vi "Actor Core.vi"(8 "error in":errorcluster caption="错误输入", 11 "服务器":refnum<class "服务器.lvclass"> caption="操作者输入") -> (0 "error out":errorcluster caption="错误输出", 3 "Actor out":refnum<class "Actor.lvclass"> caption="操作者输出")   [LabVIEW 2015, in "服务器.lvlib" / "服务器.lvclass"]
doc: "(<B>Filename</B>: Actor Framework.lvlib:Actor.lvclass:Actor Core.vi)\n\nReceives messages to the actor, reacts to them, and initiates any error handling that may shut the actor down.\n\nDescendant classes may override this VI to append parallel tasks for the actor to complete while it handles messages. Overrides use the Call Parent Method node."
uses:
  <vilib>/ActorFramework/Actor/Actor.lvclass
  <vilib>/ActorFramework/Stop Msg/Stop Msg.lvclass
  <vilib>/Instr/_visa.llb/VISA Configure Serial Port (Instr).vi
panel:
  in  "打开下位机":bool
  in  "控制中心":i32(listbox)
  in  "停止按钮":bool
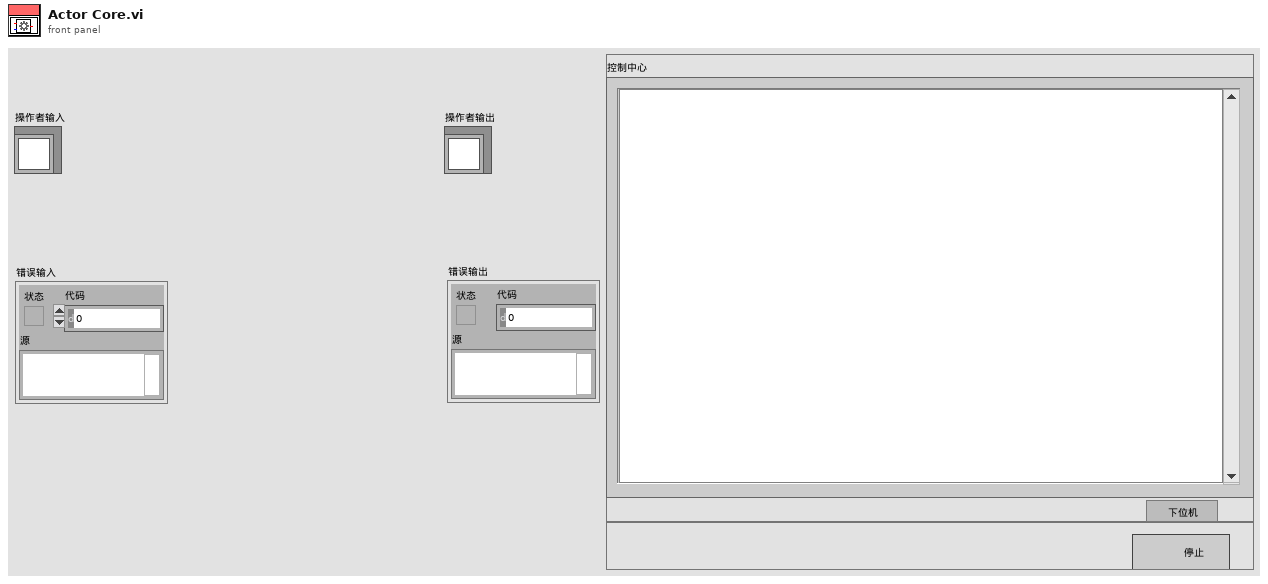
[diagram p1: front panel]
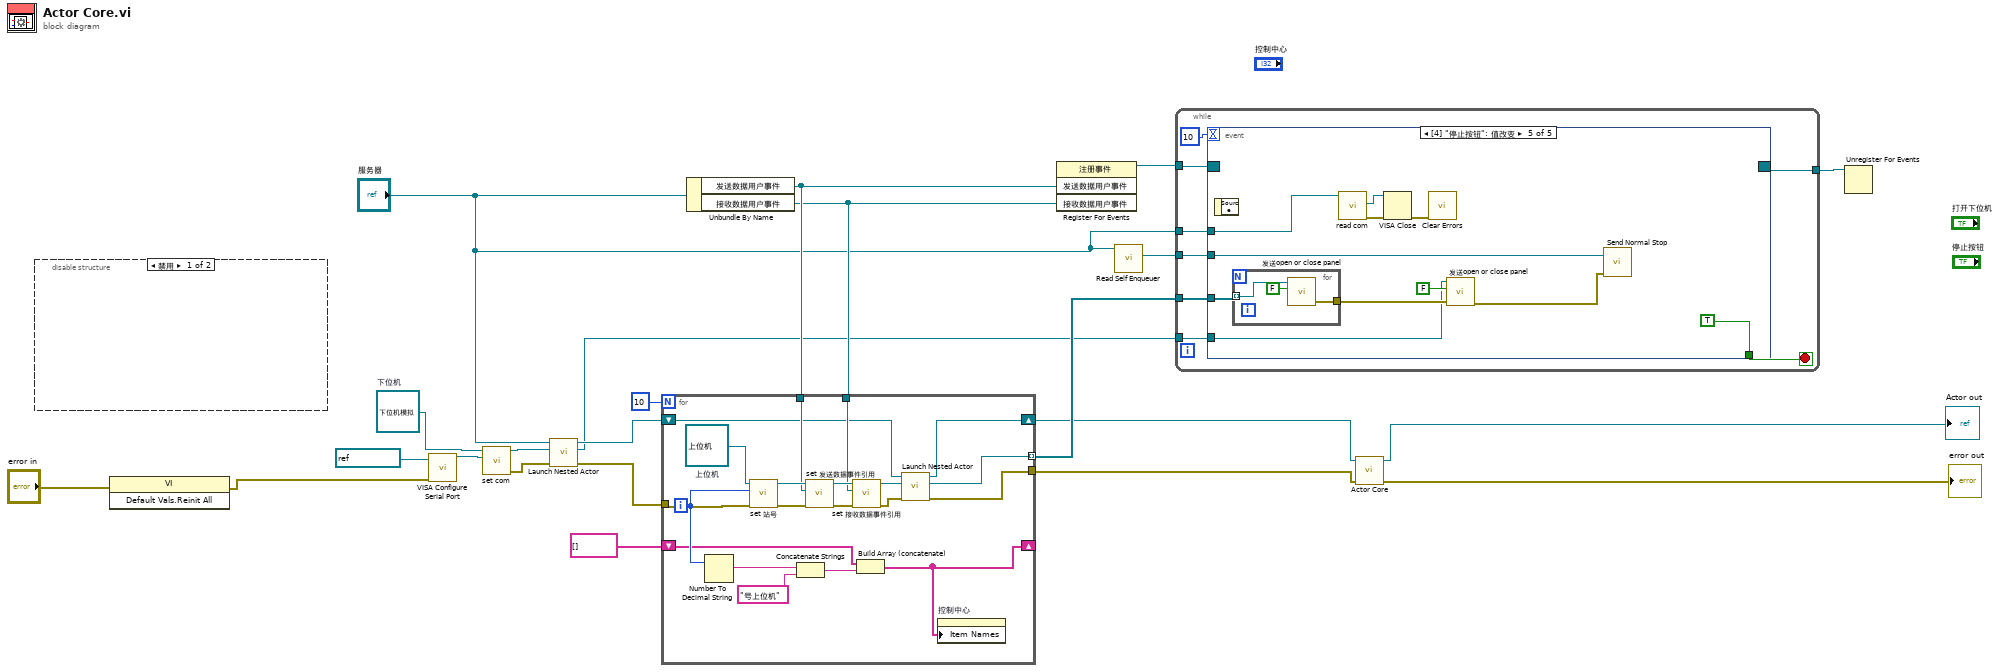
[diagram p0: block diagram]
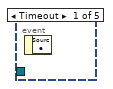
[diagram p3: hidden frame]
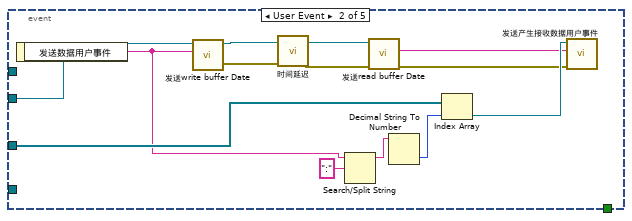
[diagram p4: hidden frame]
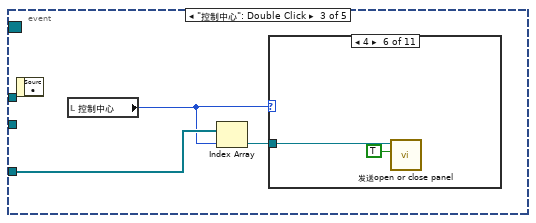
[diagram p5: hidden frame]
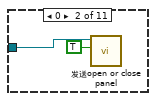
[diagram p7: hidden frame]
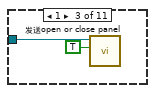
[diagram p8: hidden frame]
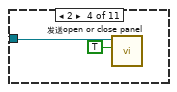
[diagram p9: hidden frame]
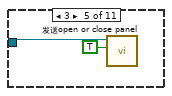
[diagram p10: hidden frame]
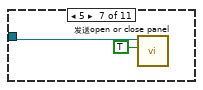
[diagram p11: hidden frame]
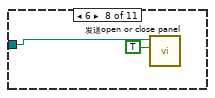
[diagram p12: hidden frame]
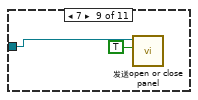
[diagram p13: hidden frame]
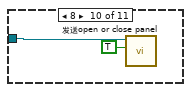
[diagram p14: hidden frame]
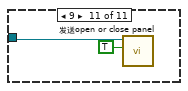
[diagram p15: hidden frame]
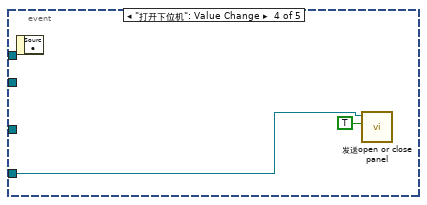
[diagram p16: hidden frame]
diagram:
  w10 = refnum<class "下位机模拟.lvclass"> refnum  # 下位机
  n1 = disable-structure shown="禁用" {
    frame Disabled {
    }
    frame Enabled {
    }
  }
  n2 = invoke class="VI" method="Default Vals.Reinit All"(error in="error in") -> (error out=w6:errorcluster)  [unwired: 2 in, 2 out]
  n3 = call-poly "VISA Configure Serial Port"("VISA resource name"=refnum<visa-resource-name> "COM29", "error in (no error)"=w6) -> ("VISA resource name out"=w7:refnum<visa-resource-name>)  [unwired: 12 in, 1 out]
  n4 = call "set com.vi"("COM"=w7, "串口参数管理 输入"=w10) -> ("error out"=w9:errorcluster, "串口参数管理 输出"=w11:refnum<class "下位机模拟.lvclass">)  [unwired: 8 in]
  n5 = call <vilib>:"Launch Nested Actor.vi"("error in (no error)"=w9, "Nested Actor"=w11, "Caller Actor in"="服务器") -> ("error out"=w4:errorcluster, "Nested Actor's Enqueuer"=w1:refnum<class "Message Enqueuer.lvclass">, "Caller Actor out"=w3:refnum<class "服务器.lvclass">)  [unwired: 6 in]
  n6 = Unbundle By Name("服务器") -> ("发送数据用户事件"=w18:refnum<user-event>, "接收数据用户事件"=w17:refnum<user-event>)
  n7 = for {
    N: 10 -> [_]
    tunnel: [w43] -> w22 mode=indexing
    tunnel: w18 -> [w36]
    tunnel: w17 -> [w35]
    tunnel: [w34] -> w13
    shift-right: [w28] -> _
    shift-left: string[] [] ("项名") -> [w27]
    tunnel: w4 -> [w26]
    shift-right: [w24] -> w2
    shift-left: w3 -> [w25]
    i -> [w30]
    w31 = refnum<class "上位机.lvclass"> refnum  # 上位机
    n8 = Number To Decimal String(number=w30) -> (decimal integer string=w29:string)  [unwired: 1 in]
    n9 = call "set 站号.vi"("error in (no error)"=w26, "站号"=w30, "上位机 输入"=w31) -> ("error out"=w39:errorcluster, "上位机 输出"=w42:refnum<class "上位机.lvclass">)  [unwired: 7 in]
    n10 = Concatenate Strings(w29, "号上位机" ("字符串")) -> (w32:string)
    n11 = call "set 发送数据事件引用.vi"("error in (no error)"=w39, "发送数据用户事件"=w36, "上位机 输入"=w42) -> ("error out"=w38:errorcluster, "上位机 输出"=w41:refnum<class "上位机.lvclass">)  [unwired: 7 in]
    n12 = call "set 接收数据事件引用.vi"("error in (no error)"=w38, "接收数据用户事件"=w35, "上位机 输入"=w41) -> ("error out"=w37:errorcluster, "上位机 输出"=w40:refnum<class "上位机.lvclass">)  [unwired: 7 in]
    n13 = Build Array (concatenate)(w27, w32) -> (w28:string[])
    n14 = call <vilib>:"Launch Nested Actor.vi"("error in (no error)"=w37, "Nested Actor"=w40, "Caller Actor in"=w25) -> ("error out"=w34:errorcluster, "Nested Actor's Enqueuer"=w43:refnum<class "Message Enqueuer.lvclass">, "Caller Actor out"=w24:refnum<class "服务器.lvclass">)  [unwired: 6 in]
    n15 = property on="控制中心" class="LstBox (严格)"("Item Names"=w28) -> ()  [unwired: 2 in, 2 out]
  }
  n16 = register-events(w18, w17) -> (reference out=w21:refnum<event-registration>)  [unwired: 2 in, 1 out]
  n17 = call <vilib>:"Read Self Enqueuer.vi"("Actor"="服务器") -> ("Self Enqueuer"=w15:refnum<class "Message Enqueuer.lvclass">)  [unwired: 10 in]
  n18 = while {
    tunnel: w22 -> [w49]
    tunnel: w21 -> [w51]
    tunnel: [w50] -> w20
    tunnel: w15 -> [w46]
    tunnel: "服务器" -> [w45]
    tunnel: w1 -> [w44]
    stop <- w48 stop-if-true
    n19 = event shown="[4] \"停止按钮\": 值改变" {
      selector: w51 -> [_ _ _ _ _]
      dyn-events: [_ _ _ _ _] -> w50
      timeout: 10 -> [_ _ _ _ _]
      tunnel: w49 -> [_ w60 w66 _ w93]
      tunnel: [_ _ _ _ TRUE] -> w48
      tunnel: w46 -> [_ w58 _ _ w95]
      tunnel: w45 -> [_ _ _ _ w94]
      tunnel: w44 -> [_ _ _ w87 w89]
      event Timeout {
        n20 = event-data() -> ()  [unwired: 1 in, 1 out]
      }
      event User Event {
        n21 = event-data() -> ("发送数据用户事件"=w57:string)  [unwired: 1 in]
        n22 = call "发送write buffer Date.vi"("写入缓冲区"=w57, "Message Enqueuer"=w58) -> ("error out"=w56:errorcluster, "Message Enqueuer out"=w55:refnum<class "Message Enqueuer.lvclass">)  [unwired: 8 in]
        n23 = call "时间延迟"("error in (no error)"=w56) -> ("error out"=w54:errorcluster)  [unwired: 10 in]
        n24 = Search/Split String(string=w57, search string/char (-)=":") -> (substring before match=w63:string)  [unwired: 1 in, 2 out]
        n25 = call "发送read buffer Date.vi"("error in (no error)"=w54, "Message Enqueuer"=w55) -> ("error out"=w53:errorcluster, "read buffer date"=w52:string)  [unwired: 7 in, 1 out]
        n26 = Decimal String To Number(string=w63) -> (number=w62:i32)  [unwired: 2 in, 1 out]
        n27 = Index Array(array=w60, index=w62) -> (element=w59:refnum<class "Message Enqueuer.lvclass">)
        n28 = call "发送产生接收数据用户事件.vi"("error in (no error)"=w53, "产生接收数据事件"=w52, "Message Enqueuer"=w59) -> ()  [unwired: 7 in, 2 out]
      }
      event "控制中心": Double Click {
        n29 = event-data() -> ()  [unwired: 1 in, 1 out]
        n30 = local read "控制中心"() -> (w65:i32)
        n31 = Index Array(array=w66, index=w65) -> (element=w64:refnum<class "Message Enqueuer.lvclass">)
        n32 = case shown="4" w65 {
          tunnel: w64 -> [_ w68 w70 w72 w73 w75 w77 w79 w81 w83 w85]
          frame Default {
          }
          frame 0 {
            n33 = call "发送open or close panel.vi"("布尔"=TRUE, "Message Enqueuer"=w68) -> ()  [unwired: 8 in, 2 out]
          }
          frame 1 {
            n34 = call "发送open or close panel.vi"("布尔"=TRUE, "Message Enqueuer"=w70) -> ()  [unwired: 8 in, 2 out]
          }
          frame 2 {
            n35 = call "发送open or close panel.vi"("布尔"=TRUE, "Message Enqueuer"=w72) -> ()  [unwired: 8 in, 2 out]
          }
          frame 3 {
            n36 = call "发送open or close panel.vi"("布尔"=TRUE, "Message Enqueuer"=w73) -> ()  [unwired: 8 in, 2 out]
          }
          frame 4 {
            n37 = call "发送open or close panel.vi"("布尔"=TRUE, "Message Enqueuer"=w75) -> ()  [unwired: 8 in, 2 out]
          }
          frame 5 {
            n38 = call "发送open or close panel.vi"("布尔"=TRUE, "Message Enqueuer"=w77) -> ()  [unwired: 8 in, 2 out]
          }
          frame 6 {
            n39 = call "发送open or close panel.vi"("布尔"=TRUE, "Message Enqueuer"=w79) -> ()  [unwired: 8 in, 2 out]
          }
          frame 7 {
            n40 = call "发送open or close panel.vi"("布尔"=TRUE, "Message Enqueuer"=w81) -> ()  [unwired: 8 in, 2 out]
          }
          frame 8 {
            n41 = call "发送open or close panel.vi"("布尔"=TRUE, "Message Enqueuer"=w83) -> ()  [unwired: 8 in, 2 out]
          }
          frame 9 {
            n42 = call "发送open or close panel.vi"("布尔"=TRUE, "Message Enqueuer"=w85) -> ()  [unwired: 8 in, 2 out]
          }
        }
      }
      event "打开下位机": Value Change {
        n43 = event-data() -> ()  [unwired: 1 in, 1 out]
        n44 = call "发送open or close panel.vi"("布尔"=TRUE, "Message Enqueuer"=w87) -> ()  [unwired: 8 in, 2 out]
      }
      event "停止按钮": Value Change {
        n45 = event-data() -> ()  [unwired: 1 in, 1 out]
        n46 = for {
          tunnel: w93 -> [w101] mode=indexing
          tunnel: [w100] -> w91
          n47 = call "发送open or close panel.vi"("布尔"=FALSE, "Message Enqueuer"=w101) -> ("error out"=w100:errorcluster)  [unwired: 8 in, 1 out]
        }
        n48 = call "read com.vi"("串口参数管理 输入"=w94) -> ("error out"=w98:errorcluster, "COM"=w97:refnum<visa-resource-name>)  [unwired: 8 in, 1 out]
        n49 = VISA Close(VISA resource name=w97, error in (no error)=w98) -> (error out=w96:errorcluster)
        n50 = call <vilib>:"Clear Errors.vi"("error in (no error)"=w96) -> ()  [unwired: 5 in, 2 out]
        n51 = call "发送open or close panel.vi"("error in (no error)"=w91, "布尔"=FALSE, "Message Enqueuer"=w89) -> ("error out"=w90:errorcluster)  [unwired: 7 in, 1 out]
        n52 = call <vilib>:"Send Normal Stop.vi"("error in (no error)"=w90, "Message Enqueuer"=w95) -> ()  [unwired: 9 in, 1 out]
      }
    }
  }
  n53 = call-parent "Actor Core.vi"("error in"=w13, "Actor in"=w2) -> ("error out"=→"error out":errorcluster, "Actor out"=→"Actor out":refnum<class "Actor.lvclass">)  [unwired: 8 in]
  n54 = Unregister For Events(event registration refnum=w20) -> ()  [unwired: 1 in, 1 out]
